vi "ex1_3c1.vi"() -> ()   [LabVIEW 2017]
uses:
  <vilib>/measure/NI_MABase.lvlib
panel:
  out "Frequency played":dbl
  in  "Delay":dbl
  in  "Amplitude":dbl
  in  "Transpose (semitones)":i8
  out "Waveform Graph":waveform(dbl)(graph)
  in  "Fs":dbl=1500.0
  in  "S no":dbl=1500.0
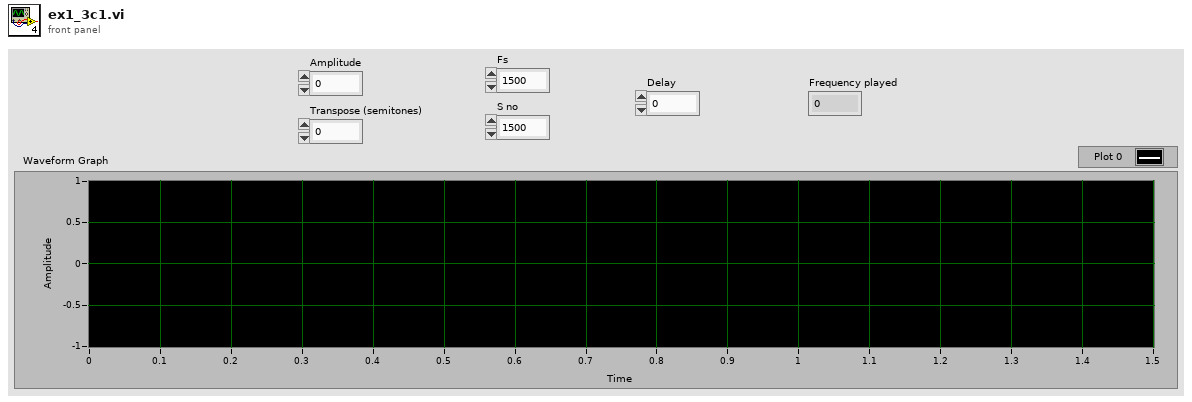
[diagram p1: front panel]
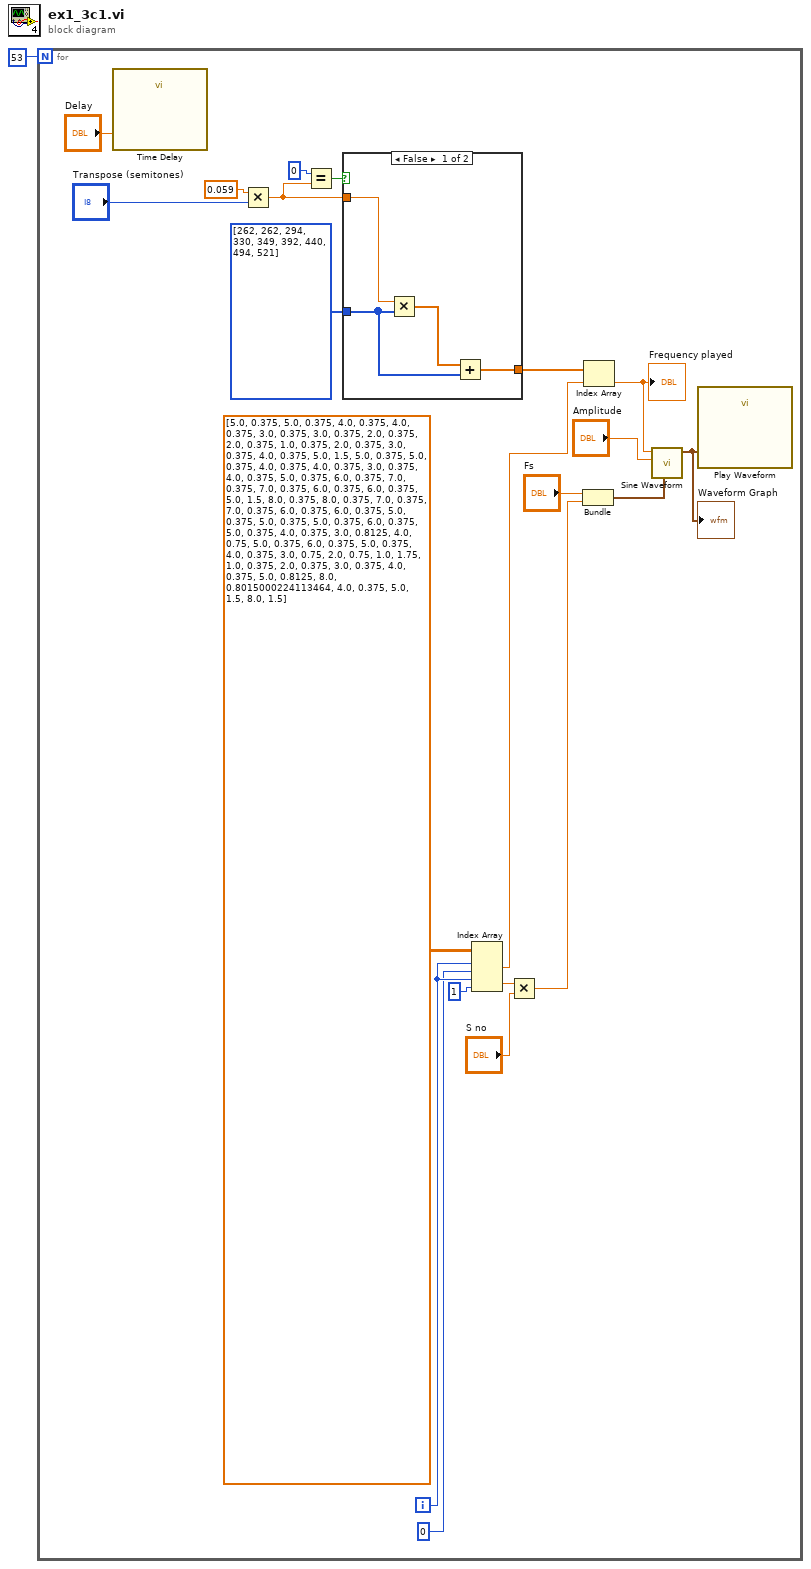
[diagram p0: block diagram]
diagram:
  n1 = for {
    N: 53 -> [_]
    i -> [w22]
    n2 = call "Time Delay"("Delay Time (s)"="Delay") -> ()  [unwired: 10 in, 1 out]
    n3 = Multiply(x=0.059, y="Transpose (semitones)") -> (x*y=w5:dbl)
    n4 = Equal?(x=0, y=w5) -> (x = y?=w6:bool)
    n5 = case shown="False" w6 {
      tunnel: i32[] [262, 262, 294, 330, 349, 392, 440, 494, 521] -> [w24 w27]
      tunnel: [w23 w27] -> w7
      tunnel: w5 -> [w26 _]
      frame False {
        n6 = Multiply(x=w26, y=w24) -> (x*y=w25:dbl[])
        n7 = Add(x=w25, y=w24) -> (x+y=w23:dbl[])
      }
      frame True {
      }
    }
    n8 = Index Array(array=sgl[][] [[5.0, 0.375], [5.0, 0.375], [4.0, 0.375], [4.0, 0.375], [3.0, 0.375], [3.0, 0.375], [2.0, 0.375], [2.0, 0.375], [1.0, 0.375], [2.0, 0.375], [3.0, 0.375], [4.0, 0.375], [5.0, 1.5], [5.0, 0.375], [5.0, 0.375], [4.0, 0.375], [4.0, 0.375], [3.0, 0.375], [4.0, 0.375], [5.0, 0.375], [6.0, 0.375], [7.0, 0.375], [7.0, 0.375], [6.0, 0.375], [6.0, 0.375], [5.0, 1.5], [8.0, 0.375], [8.0, 0.375], [7.0, 0.375], [7.0, 0.375], [6.0, 0.375], [6.0, 0.375], [5.0, 0.375], [5.0, 0.375], [5.0, 0.375], [6.0, 0.375], [5.0, 0.375], [4.0, 0.375], [3.0, 0.8125], [4.0, 0.75], [5.0, 0.375], [6.0, 0.375], [5.0, 0.375], [4.0, 0.375], [3.0, 0.75], [2.0, 0.75], [1.0, 1.75], [1.0, 0.375], [2.0, 0.375], [3.0, 0.375], [4.0, 0.375], [5.0, 0.8125], [8.0, 0.8015], [4.0, 0.375], [5.0, 1.5], [8.0, 1.5]], index (row) #1=w22, index (col) #1=0, index (row) #2=w22, index (col) #2=1) -> (element #1=w19:sgl, element #2=w15:sgl)
    n9 = Multiply(x=w15, y="S no") -> (x*y=w16:dbl)
    n10 = Bundle "Bundle"("Fs"="Fs", w16) -> (w14:cluster{"Fs":dbl, dbl})  [unwired: 1 in]
    n11 = Index Array(array=w7, index=w19) -> (element=w2:dbl)
    "Frequency played" <- w2
    n12 = call <vilib>:"Sine Waveform.vi"("sampling info"=w14, "amplitude"="Amplitude", "frequency"=w2) -> ("signal out"=w17:waveform(dbl))  [unwired: 7 in, 1 out]
    "Waveform Graph" <- w17
    n13 = call "Play Waveform"("Data"=w17) -> ()  [unwired: 18 in, 1 out]
  }
